vi "Add Information Channels.vi"(8 "error in (no error)":errorcluster, 11 "Node Ptr":u64) -> (0 "error out":errorcluster, 3 "Parent Ref out":T1 format="%.0x")   [LabVIEW 2019, in "Protection and Counter Addon System Explorer.lvlib"]
uses:
  <vilib>/NI VeriStand/Custom Device API/Custom Device Item Ref.ctl
  <vilib>/NI VeriStand/Custom Device API/Custom Device Channel.ctl
  <vilib>/NI VeriStand/Custom Device API/Custom Device Channel Type.ctl
  Addon Shared/SubVIs/GUID Lookup.vi
  Protection and Counter Addon System Explorer.lvlib
  <vilib>/NI VeriStand/Custom Device API/Custom Device API.lvlib
  <vilib>/NI/NI VeriStand Advanced SysDef API/SysDef API/Advanced System Definition.lvlib
  Addon Shared/Protection and Counter Addon Shared.lvlib
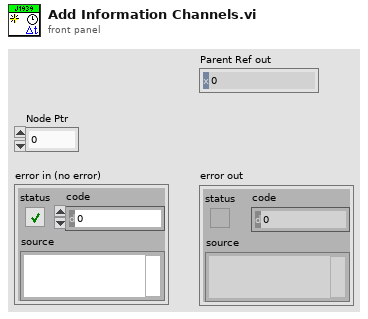
[diagram p1: front panel]
types:
  T1 = typedef "Custom Device API.lvlib/Custom Device Item Ref.ctl" = u64
  T2 = typedef "Custom Device API.lvlib/Custom Device Channel.ctl" = cluster{"Type":T3, "Units":string, "Default Value":dbl, "Faultable":bool, "Scalable":bool}
  T3 = typedef "Custom Device API.lvlib/Custom Device Channel Type.ctl" = enum16{"Input", "Output"}
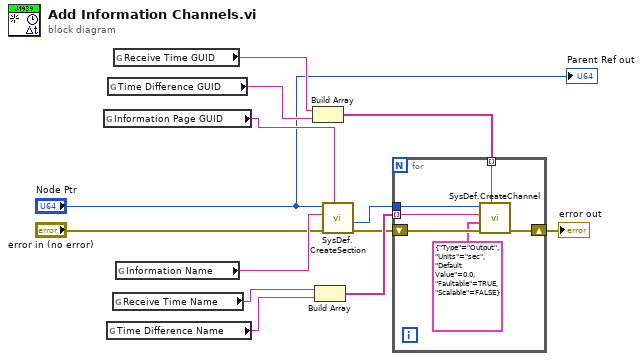
[diagram p0: block diagram]
diagram:
  n1 = global read "GUID Lookup.vi" "Information Page GUID"() -> (w7:string)
  n2 = global read "GUID Lookup.vi" "Time Difference Name"() -> (w4:string)
  n3 = global read "GUID Lookup.vi" "Time Difference GUID"() -> (w8:string)
  n4 = global read "GUID Lookup.vi" "Receive Time Name"() -> (w5:string)
  n5 = global read "GUID Lookup.vi" "Receive Time GUID"() -> (w9:string)
  n6 = global read "GUID Lookup.vi" "Information Name"() -> (w6:string)
  n7 = Build Array(w9, w8) -> (w13:string[])
  n8 = Build Array(w5, w4) -> (w12:string[])
  n9 = call <vilib>:"SysDef.CreateSection.vi"("GUID"=w7, "error in (no error)"="error in (no error)", "Name"=w6, "nodeID"="Node Ptr") -> ("error out"=w1:errorcluster, "New NodeID"=w10:u64)  [unwired: 4 in, 2 out]
  n10 = for {
    tunnel: w10 -> [w18]
    shift-right: [w17] -> w11
    shift-left: w1 -> [w19]
    tunnel: w13 -> [w15] mode=indexing
    tunnel: w12 -> [w14] mode=indexing
    n11 = call <vilib>:"SysDef.CreateChannel.vi"("GUID"=w15, "error in (no error)"=w19, "Channel"=T2 {"Type"=enum."Output", "Units"="sec", "Default Value"=0.0, "Faultable"=TRUE, "Scalable"=FALSE}, "Name"=w14, "nodeID"=w18) -> ("error out"=w17:errorcluster)  [unwired: 3 in, 3 out]
  }
  "error out" <- w11
  "Parent Ref out" <- "Node Ptr"
